vi "testWriter.vi"() -> ()   [LabVIEW 2013]
uses:
  RIO-OCU_Comm/NetworkStreams/Writer/NetworkStreamWriter.lvclass
panel:
  in  "error in (no error)":errorcluster
  out "Connected?":bool
  in  "stop":bool
  in  "boat speed":dbl
  out "error out":errorcluster
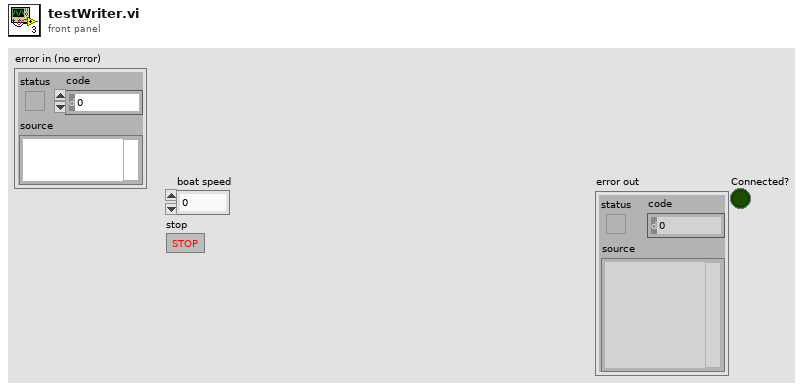
[diagram p1: front panel]
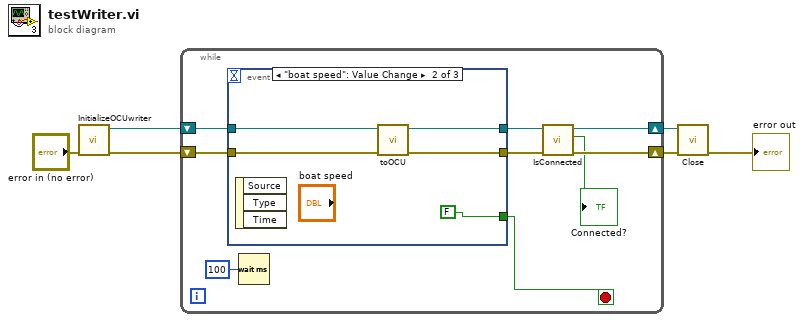
[diagram p0: block diagram]
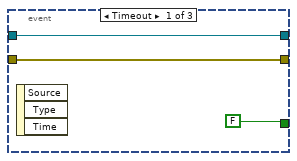
[diagram p2: hidden frame]
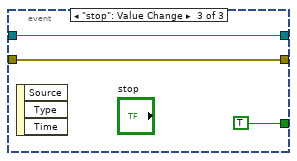
[diagram p3: hidden frame]
diagram:
  n1 = call "InitializeOCUwriter.vi"("error in (no error)"="error in (no error)") -> ("error out"=w6:errorcluster, "NetworkStreamWriter out"=w5:refnum<class "NetworkStreamWriter.lvclass">)  [unwired: 9 in]
  n2 = while {
    shift-right: [w10] -> w2
    shift-left: w5 -> [w14]
    shift-right: [w12] -> w4
    shift-left: w6 -> [w15]
    stop <- w7 stop-if-true
    n3 = event shown="[1] \"boat speed\": Value Change" {
      selector: _ -> [_ _ _]
      dyn-events: _ -> [_ _ _]
      timeout: _ -> [_ _ _]
      tunnel: w15 -> [w17 w20 w24]
      tunnel: w14 -> [w18 w21 w25]
      tunnel: [w18 w23 w25] -> w11
      tunnel: [w17 w22 w24] -> w13
      tunnel: [FALSE FALSE TRUE] -> w7
      event Timeout {
        n4 = event-data() -> ()  [unwired: 1 in, 3 out]
      }
      event "boat speed": Value Change {
        n5 = event-data() -> ()  [unwired: 1 in, 3 out]
        n6 = call "toOCU.vi"("error in (no error)"=w20, "NetworkStreamWriter in"=w21) -> ("error out"=w22:errorcluster, "NetworkStreamWriter out"=w23:refnum<class "NetworkStreamWriter.lvclass">)  [unwired: 8 in]
      }
      event "stop": Value Change {
        n7 = event-data() -> ()  [unwired: 1 in, 3 out]
      }
    }
    n8 = Wait (ms)(milliseconds to wait=u32 100) -> ()  [unwired: 1 out]
    n9 = call "IsConnected.vi"("error in (no error)"=w13, "NetworkStreamWriter in"=w11) -> ("error out"=w12:errorcluster, "Connected?"=→"Connected?":bool, "NetworkStreamWriter out"=w10:refnum<class "NetworkStreamWriter.lvclass">)  [unwired: 7 in]
  }
  n10 = call "Close.vi"("error in (no error)"=w4, "NetworkStreamWriter in"=w2) -> ("error out"=→"error out":errorcluster)  [unwired: 9 in]
